vi "Override Joystick.vi"(2 "JoystickDevRef":T1) -> (10 "axis 1 (x)":dbl, 13 "Top":bool, 14 "axis 2 (y)":dbl, 15 "Middle":bool, 17 "Floor":bool, 18 "Drive Override":bool, 19 "Invert":bool, 20 "axis 3 (throttle)":dbl, 22 "X override":bool, 24 "Y override":bool, 26 "Set RPM":bool)   [LabVIEW 2011]
uses:
  <vilib>/Rock Robotics/WPI/Joystick/WPI_JoystickDevRef.ctl
  <vilib>/Rock Robotics/WPI/Joystick/WPI_JoystickDeviceEnum.ctl
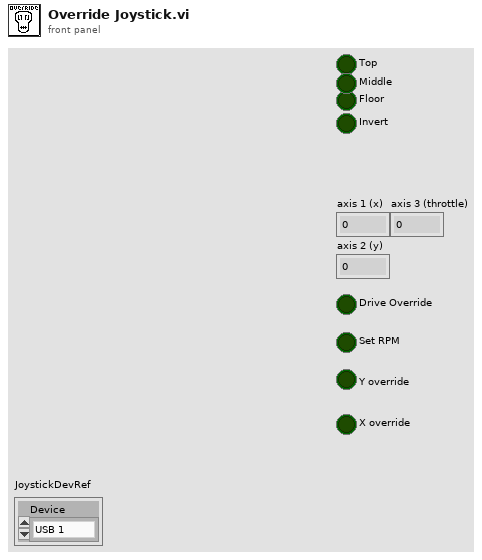
[diagram p1: front panel]
types:
  T1 = typedef "WPI_JoystickDevRef.ctl" = cluster{"Device":T2}
  T2 = typedef "WPI_JoystickDeviceEnum.ctl" = enum16{"USB 1", "USB 2", "USB 3", "USB 4", "Kinect 1", "Kinect 2"}
  T3 = typedef "WPI_JoystickButtonState.ctl" = cluster{"Button 1":bool, "Button 2":bool, "Button 3":bool, "Button 4":bool, "Button 5":bool, "Button 6":bool, "Button 7":bool, "Button 8":bool, "Button 9":bool, "Button 10":bool, "Button 11":bool, "Button 12":bool}
  T4 = cluster{"axis 1 (x)":dbl, "axis 2 (y)":dbl, "axis 3 (throttle)":dbl, "axis 4":dbl, "axis 5":dbl, "axis 6":dbl}
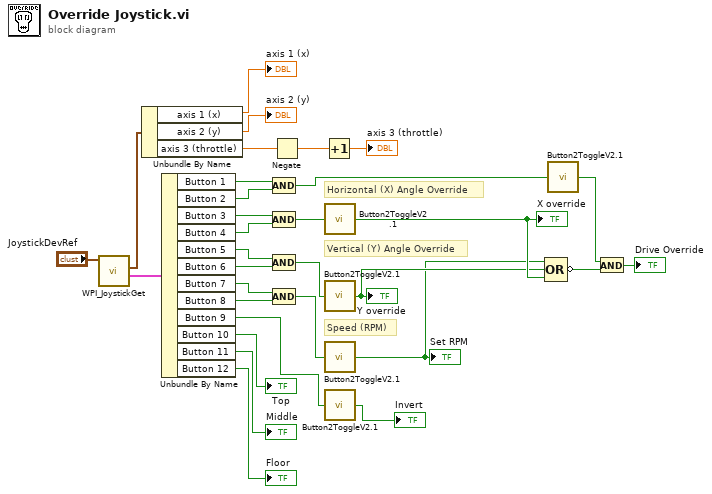
[diagram p0: block diagram]
diagram:
  # "Speed (RPM)"
  # "Vertical (Y) Angle Override"
  # "Horizontal (X) Angle Override"
  n1 = call <vilib>:"WPI_JoystickGet.vi"("JoystickDevRef"="JoystickDevRef") -> ("Buttons"=w29:T3, "Axes"=w30:T4)  [unwired: 4 in, 1 out]
  n2 = Unbundle By Name(w30) -> ("axis 1 (x)"=→"axis 1 (x)":dbl, "axis 2 (y)"=→"axis 2 (y)":dbl, "axis 3 (throttle)"=w16:dbl)
  n3 = Unbundle By Name(w29) -> ("Button 1"=w28:bool, "Button 2"=w27:bool, "Button 3"=w25:bool, "Button 4"=w24:bool, "Button 5"=w26:bool, "Button 6"=w23:bool, "Button 7"=w22:bool, "Button 8"=w21:bool, "Button 9"=w2:bool, "Button 10"=→"Top":bool, "Button 11"=→"Middle":bool, "Button 12"=→"Floor":bool)
  n4 = Negate(x=w16) -> (-x=w15:dbl)
  n5 = Compound Arithmetic op=AND(w28, w27) -> (w13:bool)
  n6 = Compound Arithmetic op=AND(w25, w24) -> (w11:bool)
  n7 = Compound Arithmetic op=AND(w26, w23) -> (w9:bool)
  n8 = Compound Arithmetic op=AND(w22, w21) -> (w7:bool)
  n9 = Increment(x=w15) -> (x+1=→"axis 3 (throttle)":dbl)
  n10 = call "Button2ToggleV2.1.vi"("a"=w11) -> ("Result(clone)"=w10:bool)
  "X override" <- w10
  n11 = call "Button2ToggleV2.1.vi"("a"=w9) -> ("Result(clone)"=w8:bool)
  "Y override" <- w8
  n12 = call "Button2ToggleV2.1.vi"("a"=w7) -> ("Result(clone)"=w3:bool)
  "Set RPM" <- w3
  n13 = call "Button2ToggleV2.1.vi"("a"=w2) -> ("Result(clone)"=→"Invert":bool)
  n14 = Compound Arithmetic op=OR(w3, w8, w10) -> (invert w20:bool)
  n15 = call "Button2ToggleV2.1.vi"("a"=w13) -> ("Result(clone)"=w12:bool)
  n16 = And(x=w12, y=w20) -> (x .and. y?=→"Drive Override":bool)
